vi "Actor Core.vi"(8 "error in":errorcluster, 11 "AssertEngine in":refnum<class "AssertEngine.lvclass">) -> (0 "error out":errorcluster, 3 "Actor out":refnum<class "Actor.lvclass">)   [LabVIEW 2016, in "AssertEngine.lvlib" / "AssertEngine.lvclass"]
doc: "(<B>Filename</B>: Actor Framework.lvlib:Actor.lvclass:Actor Core.vi)\n\nReceives messages to the actor, reacts to them, and initiates any error handling that may shut the actor down.\n\nDescendant classes may override this VI to append parallel tasks for the actor to complete while it handles messages. Overrides use the Call Parent Method node."
uses:
  AssertEngine.lvclass
  C:/Program Files/National Instruments/LabVIEW 2016/vi.lib/ActorFramework/Actor/Actor.lvclass
  <vilib>/ActorFramework/Actor/Actor.lvclass
  UserInterface/UserInterface/UserInterface.lvclass
  AssertEngine.lvclass/AssertEngine.ctl
  UserInterface/UserInterface Messages/Change Panel State Msg/Change Panel State Msg.lvclass/Change Panel State Msg.ctl
  <vilib>/ActorFramework/Message Enqueuer/Message Enqueuer.lvclass/Message Enqueuer.ctl
  <vilib>/ActorFramework/Message Enqueuer/Enqueue.vi
  UserInterface/UserInterface Messages/Change Panel State Msg/Change Panel State Msg.lvclass
  C:/Program Files/National Instruments/LabVIEW 2016/vi.lib/ActorFramework/Message/Message.lvclass
  <vilib>/ActorFramework/Message Priority Queue/Priority Enqueue.vi
  AssertEngine.lvlib
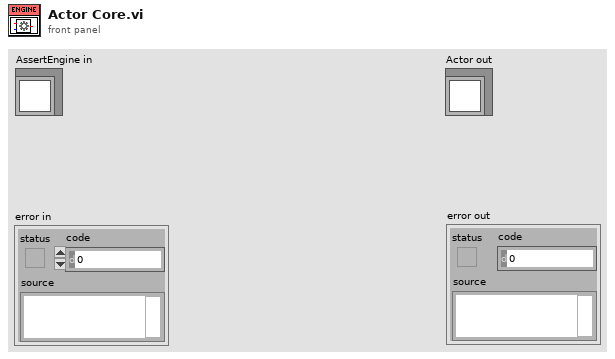
[diagram p1: front panel]
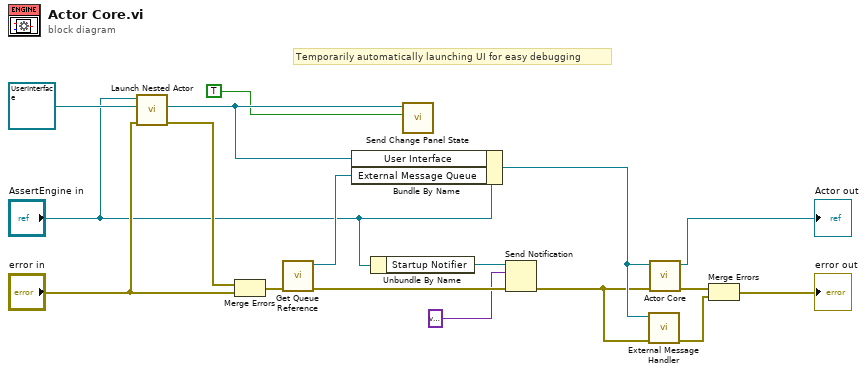
[diagram p0: block diagram]
diagram:
  # "Temporarily automatically launching UI for easy debugging"
  n1 = call <vilib>:"Launch Nested Actor.vi"("error in (no error)"="error in", "Nested Actor"=refnum<class "UserInterface.lvclass"> refnum ("UserInterface.lvlib:UserInterface.lvclass"), "Caller Actor in"="AssertEngine in") -> ("error out"=w12:errorcluster, "Nested Actor's Enqueuer"=w11:refnum<class "Message Enqueuer.lvclass">)  [unwired: 6 in, 1 out]
  n2 = Merge Errors(w12, "error in") -> (w13:errorcluster)
  n3 = call "Get Queue Reference.vi"("error in (no error)"=w13) -> ("error out"=w7:errorcluster, "Message Queue"=w9:refnum<queue>)  [unwired: 8 in, 1 out]
  n4 = Bundle By Name(cluster="AssertEngine in", "User Interface"=w11, "External Message Queue"=w9) -> (w8:refnum<class "AssertEngine.lvclass">)
  n5 = Unbundle By Name("AssertEngine in") -> ("Startup Notifier"=w2:refnum<notifier>)
  n6 = call "Send Change Panel State.vi"("Open/Close"=TRUE, "Message Enqueuer"=w11) -> ()  [unwired: 8 in, 2 out]
  n7 = Send Notification(notification=variant, notifier=w2, error in (no error)=w7) -> (error out=w3:errorcluster)  [unwired: 1 out]
  n8 = call "External Message Handler.vi"("error in (no error)"=w3, "AssertEngine in"=w8) -> ("error out"=w5:errorcluster)  [unwired: 9 in]
  n9 = call-parent "Actor Core.vi"("error in"=w3, "Actor in"=w8) -> ("error out"=w17:errorcluster, "Actor out"=→"Actor out":refnum<class "Actor.lvclass">)  [unwired: 8 in]
  n10 = Merge Errors(w17, w5) -> (→"error out":errorcluster)
